vi "_malloc.vi"(6 "DT":T1, 7 "Copies Count(1)":i32=1, 9 "String Attribute":string, 10 "error in (no error)":errorcluster, 11 "String":string) -> (2 "error out":errorcluster, 3 "MDPtr DVR":refnum<data-value>)   [LabVIEW 2017, in "MDPtr.lvlib"]
uses:
  MDPtr.lvlib
  MDPtr TypeDef/MDPtr DataFrame-Memory.ctl
  MDPtr TypeDef/MDPtr DataFrame-Common.ctl
  <vilib>/Utility/Data Type/Type Definitions/Data Type.ctl
  <vilib>/Utility/Data Type/NI_Data Type.lvlib
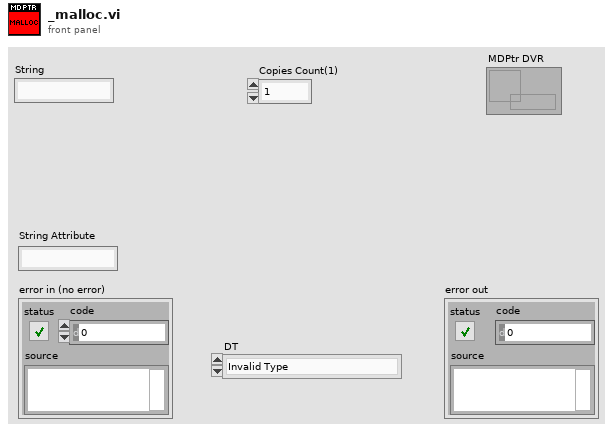
[diagram p1: front panel]
types:
  T1 = typedef "NI_Data Type.lvlib/Data Type.ctl" = enum8{"Invalid Type", "Void", "I8", "I16", "I32", "I64", "U8", "U16", "U32", "U64", "Single Float", "Double Float", "Extended Float", "Single Complex", "Double Complex", "Extended Complex", "Enum U8", "Enum U16", "Enum U32", "Enum U64", "Single Float With Unit", "Double Float With Unit", "Extended Float With Unit", "Single Complex with Unit", "Double Complex with Unit", "Extended Complex with Unit", "Boolean", "String", "Path", "Picture", "Tag", "Array", "Cluster", "Variant", "LV Variant", "Waveform", "Timestamp", "Digital Waveform", "Digital Data", "ExpressData", "Refnum", "External Data", "VI", "Poly VI", "LabVIEW Class Instance", "Fixed Point"}
  T2 = typedef "MDPtr.lvlib/MDPtr DataFrame-Memory.ctl" = cluster{"Common":T3, "DVR":refnum<data-value>}
  T3 = typedef "MDPtr.lvlib/MDPtr DataFrame-Common.ctl" = cluster{"Data Type":T1, "Copy Count":i32, "String Attribute":string, "Cache Length":i32, "Data Length":i32}
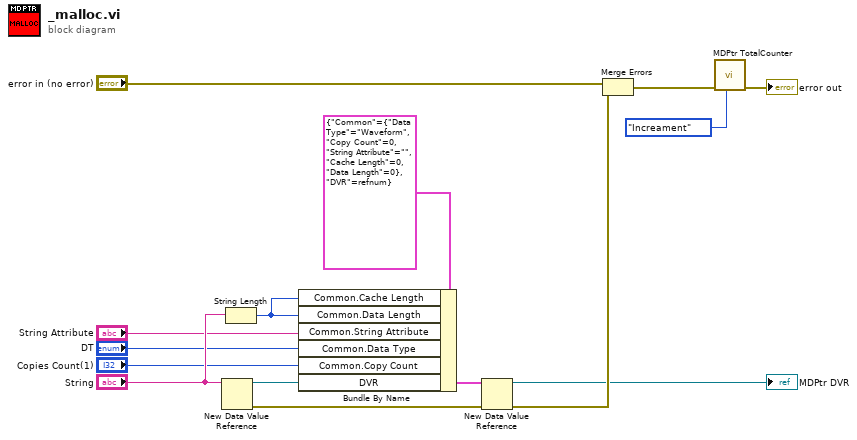
[diagram p0: block diagram]
diagram:
  n1 = New Data Value Reference(data value="String") -> (data value reference=w8:refnum<data-value>, error out=w10:errorcluster)  [unwired: 1 in]
  n2 = String Length(string="String") -> (length=w6:i32)
  n3 = Bundle By Name(cluster=T2 {"Common"={"Data Type"=enum."Waveform", "Copy Count"=0, "String Attribute"="", "Cache Length"=0, "Data Length"=0}, "DVR"=refnum} ("DataFrame-String"), "Common.Cache Length"=w6, "Common.Data Length"=w6, "Common.String Attribute"="String Attribute", "Common.Data Type"="DT", "Common.Copy Count"="Copies Count(1)", "DVR"=w8) -> (w11:T2)
  n4 = New Data Value Reference(data value=w11, error in=w10) -> (data value reference=→"MDPtr DVR":refnum<data-value>, error out=w4:errorcluster)
  n5 = Merge Errors("error in (no error)", w4) -> (w3:errorcluster)
  n6 = call "MDPtr TotalCounter.vi"("Oper(Get)"=enum16{"GET", "Increament", "decreament"}."Increament", "error in (no error)"=w3) -> ("error out"=→"error out":errorcluster)  [unwired: 8 in, 1 out]
